vi "Timestamp.vi"(8 "error in (no error)":errorcluster, 10 "First Time":timestamp, 11 "Paquetes Disponibles in":refnum<class "Paquetes Disponibles.lvclass">) -> (0 "error out":errorcluster, 3 "Paquetes Disponibles out":refnum<class "Paquetes Disponibles.lvclass">)   [LabVIEW 2020, in "Paquetes Disponibles.lvlib" / "Paquetes Disponibles.lvclass"]
uses:
  Paquetes Disponibles.lvclass
  Paquetes Disponibles.lvclass/Paquetes Disponibles.ctl
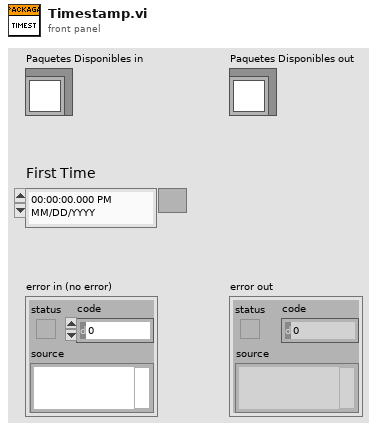
[diagram p1: front panel]
types:
  T1 = typedef "LVDateTimeRec.ctl" = cluster{"fractional second":dbl, "second":i32, "minute":i32, "hour":i32, "day of month":i32, "month":i32, "year":i32, "day of week":i32, "day of year":i32, "DST":i32}
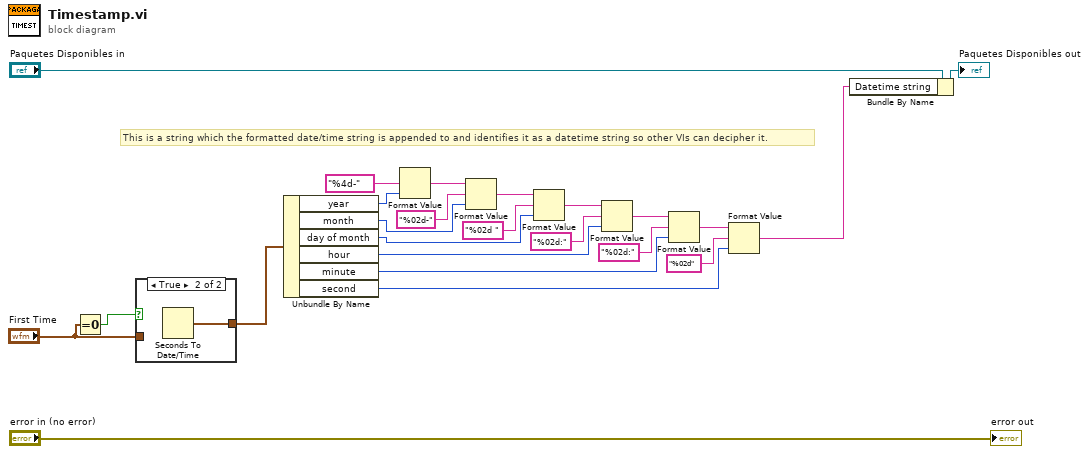
[diagram p0: block diagram]
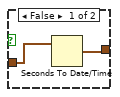
[diagram p2: hidden frame]
diagram:
  # "This is a string which the formatted date/time string is appended to and identifies it as a datetime string so other VIs can decipher it."
  n1 = Equal To 0?(x="First Time") -> (x = 0?=w21:bool)
  n2 = case shown="True" w21 {
    tunnel: [w25 w27] -> w20
    tunnel: "First Time" -> [w26 _]
    frame False {
      n3 = Seconds To Date/Time(time stamp (now)=w26) -> (date time rec=w25:T1)  [unwired: 1 in]
    }
    frame True {
      n4 = Seconds To Date/Time() -> (date time rec=w27:T1)  [unwired: 2 in]
    }
  }
  n5 = Unbundle By Name(w20) -> ("year"=w15:i32, "month"=w16:i32, "day of month"=w17:i32, "hour"=w3:i32, "minute"=w6:i32, "second"=w7:i32)
  n6 = Format Value(format string="%4d-", value (0)=w15) -> (output string=w12:string)  [unwired: 1 in]
  n7 = Format Value(string ("")=w12, format string="%02d-", value (0)=w16) -> (output string=w13:string)
  n8 = Format Value(string ("")=w13, format string="%02d ", value (0)=w17) -> (output string=w14:string)
  n9 = Format Value(string ("")=w14, format string="%02d:", value (0)=w3) -> (output string=w4:string)
  n10 = Format Value(string ("")=w4, format string="%02d:", value (0)=w6) -> (output string=w5:string)
  n11 = Format Value(string ("")=w5, format string="%02d", value (0)=w7) -> (output string=w1:string)
  n12 = Bundle By Name(cluster="Paquetes Disponibles in", "Datetime string"=w1) -> (→"Paquetes Disponibles out":refnum<class "Paquetes Disponibles.lvclass">)
  "error out" <- "error in (no error)"
